vi "Settings.vi"(8 "Error In":errorcluster, 11 "CAD Dispense in":refnum<class "CAD Dispense.lvclass">) -> (0 "Error Out":errorcluster, 3 "CAD Dispense out":refnum<class "CAD Dispense.lvclass">)   [LabVIEW 2020, in "CAD Dispense.lvclass"]
uses:
  CAD Dispense.lvclass
  C:/Users/hep/Documents/CMU gantry/Classes/Routine/Dispense/Dispense.lvclass
  CAD Dispense.lvclass/CAD Dispense.ctl
  Dispense.lvclass/Dispense.ctl
  Write Tip Height.vi
  Dispense.lvclass
panel:
  in  "Time?":bool
  in  "Pattern":u16(ring) items=["Circle 5", "Circle 6", "Le Cercle Deux", "Le Cercle Quatre", "Le Cercle Un", "Le CercleTre", "Reasonable Glue", "Reasonable Glue 2", "Reasonable Glue 3", "Reasonable Glue 4", "Reasonable Glue 5", "Reasonable Glue 6"]
  in  "Glue Speed":i32=15
  in  "Move Speed":i32=30
  in  "Pressure (psi)":i64=70
  in  "Tip Height":dbl=0.25 format="%#_13g"
  in  "Submit":bool=TRUE
  # "CAD Dispense"
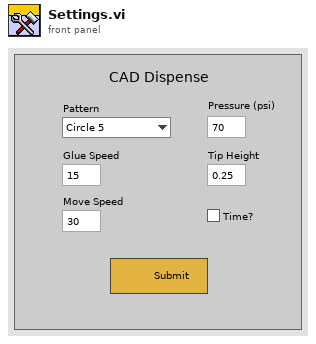
[diagram p1: front panel]
types:
  T1 = typedef "File Paths.ctl" = cluster{"Glue Pattern Folder":path, "Carrier Tray Folder":path, "Pick Up Tool Fixture Folder":path, "Components Folder":path, "Bellows Tool Offset.txt":path, "Pick Up Tool Offset.txt":path, "Dispense Tip Offset.txt":path, "Log Files":path}
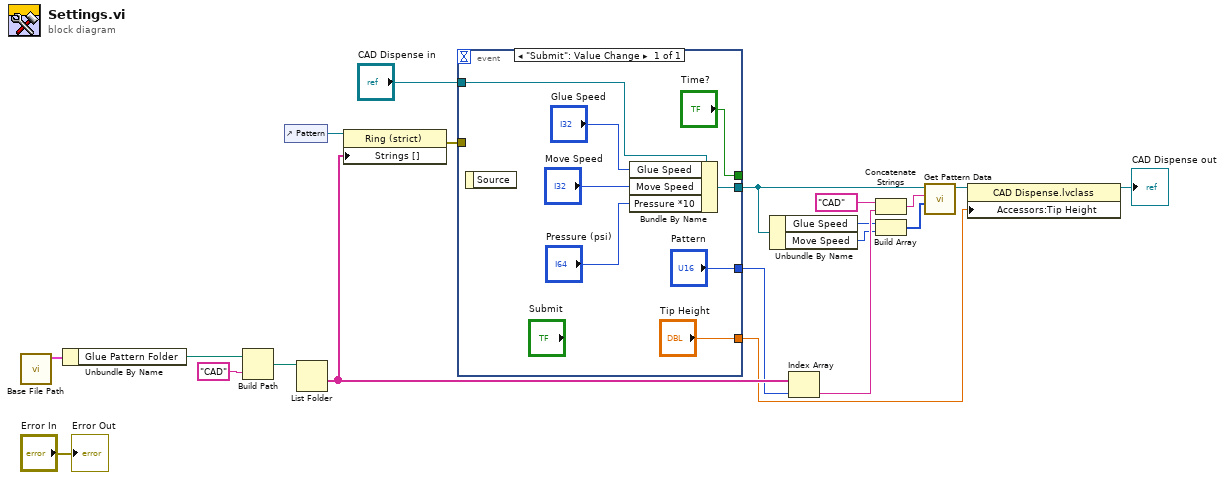
[diagram p0: block diagram]
diagram:
  n1 = call "Base File Path.vi"() -> ("Paths Out"=w19:T1)  [unwired: 11 in]
  n2 = Unbundle By Name(w19) -> ("Glue Pattern Folder"=w18:path)
  n3 = Build Path(base path=w18, name or relative path="CAD") -> (appended path=w11:path)
  n4 = control-ref of="Pattern"() -> (w16:refnum<vi>)
  n5 = List Folder(path=w11) -> (folder names=w14:string[])  [unwired: 3 in, 3 out]
  n6 = property class="Ring (strict)"(reference=w16, "Strings []"=w14) -> (error out=w15:errorcluster)  [unwired: 1 in, 1 out]
  n7 = event shown="[0] \"Submit\": Value Change" {
    selector: _ -> [_]
    dyn-events: _ -> [_]
    timeout: _ -> [_]
    tunnel: "CAD Dispense in" -> [w28]
    tunnel: [w26] -> w2
    tunnel: w15 -> [_]
    tunnel: ["Pattern"] -> w13
    tunnel: ["Time?"] -> _
    tunnel: ["Tip Height"] -> w9
    event "Submit": Value Change {
      n8 = event-data() -> ()  [unwired: 1 in, 1 out]
      n9 = Bundle By Name(cluster=w28, "Glue Speed"="Glue Speed", "Move Speed"="Move Speed", "Pressure *10"="Pressure (psi)") -> (w26:refnum<class "CAD Dispense.lvclass">)
    }
  }
  n10 = Unbundle By Name(w2) -> ("Glue Speed"=w5:i32, "Move Speed"=w4:i32)
  n11 = Index Array(array=w14, index=w13) -> (element=w7:string)
  n12 = Concatenate Strings("CAD", w7) -> (w6:string)
  n13 = Build Array(w5, w4) -> (w3:i32[])
  n14 = call "Get Pattern Data.vi"("File Name"=w3, "Folder Name"=w6, "Dispense.lvclass"=w2) -> ("Dispense Out"=w1:refnum<class "CAD Dispense.lvclass">)  [unwired: 8 in]
  n15 = property class="CAD Dispense.lvclass"(reference=w1, "Accessors:Tip Height"=w9) -> (reference out=→"CAD Dispense out":refnum<class "CAD Dispense.lvclass">)  [unwired: 1 in, 1 out]
  "Error Out" <- "Error In"
